vi "Global VI for Localized Text.vi"() -> ()   [LabVIEW 2020, in "NI_TDMS File Viewer.lvlib"]
uses:
  <vilib>/Utility/TDMS File Viewer/NI_TDMS File Viewer.lvlib
panel:
  in  "False":string="false"
  in  "True":string="true"
  in  "pattern label tdms":string="TDMS File"
  in  "prompt tdms":string="Select a TDMS File"
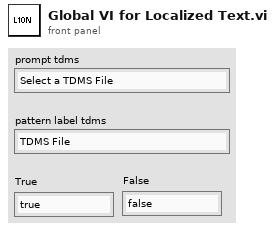
[diagram p1: front panel]
diagram:
